vi "cvt type to tag bus type.vi"(11 "cvt type":T1) -> (3 "Data Type":T2)   [LabVIEW 2013, in "CVT configuration.lvclass"]
uses:
  CVT configuration.lvclass
  <vilib>/NI/Tag Bus/tag/Data Type.ctl
  <vilib>/NI/Current Value Table/Type Defs/Data Types.ctl
  <vilib>/NI/Tag Bus/tag/tag descriptor.lvclass
  <vilib>/NI/Current Value Table/Current Value Table.lvlib
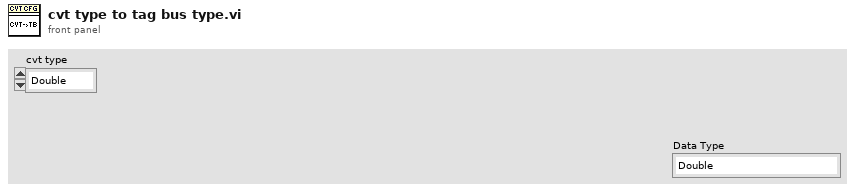
[diagram p1: front panel]
types:
  T1 = typedef "Current Value Table.lvlib/Data Types.ctl" = enum16{"Double", "Single", "I64", "I32", "I16", "I8", "U64", "U32", "U16", "U8", "String", "Boolean", "Array of U8", "Array of U16", "Array of U32", "Array of U64", "Array of I64", "Array of I32", "Array of I16", "Array of I8", "Array of Double", "Array of Single", "Array of Boolean", "Array of String"}
  T2 = typedef "tag bus.lvlib/tag descriptor.lvclass/Data Type.ctl" = enum16{"Double", "Single", "I64", "I32", "I16", "I8", "U64", "U32", "U16", "U8", "Boolean", "String", "Array of Double", "Array of Single", "Array of I64", "Array of I32", "Array of I16", "Array of I8", "Array of U64", "Array of U32", "Array of U16", "Array of U8", "Array of Boolean", "Array of String"}
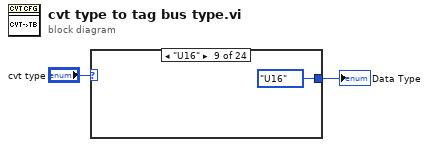
[diagram p0: block diagram]
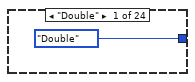
[diagram p2: hidden frame]
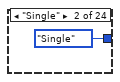
[diagram p3: hidden frame]
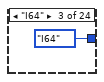
[diagram p4: hidden frame]
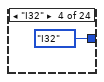
[diagram p5: hidden frame]
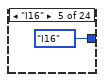
[diagram p6: hidden frame]
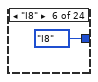
[diagram p7: hidden frame]
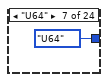
[diagram p8: hidden frame]
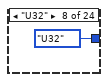
[diagram p9: hidden frame]
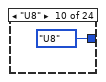
[diagram p10: hidden frame]
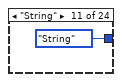
[diagram p11: hidden frame]
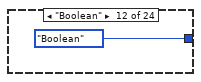
[diagram p12: hidden frame]
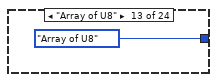
[diagram p13: hidden frame]
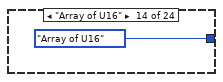
[diagram p14: hidden frame]
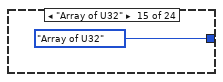
[diagram p15: hidden frame]
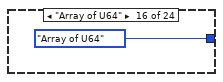
[diagram p16: hidden frame]
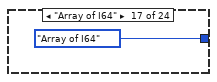
[diagram p17: hidden frame]
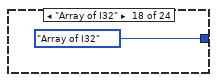
[diagram p18: hidden frame]
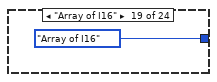
[diagram p19: hidden frame]
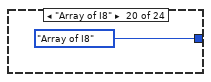
[diagram p20: hidden frame]
diagram:
  n1 = case shown="\"U16\"" "cvt type" {
    tunnel: [Data_Type."Double" ("Expected Type") Data_Type."Single" ("Expected Type") Data_Type."I64" ("Expected Type") Data_Type."I32" ("Expected Type") Data_Type."I16" ("Expected Type") Data_Type."I8" ("Expected Type") Data_Type."U64" ("Expected Type") Data_Type."U32" ("Expected Type") Data_Type."U16" ("Expected Type") Data_Type."U8" ("Expected Type") Data_Type."String" ("Expected Type") Data_Type."Boolean" ("Expected Type") Data_Type."Array of U8" ("Expected Type") Data_Type."Array of U16" ("Expected Type") Data_Type."Array of U32" ("Expected Type") Data_Type."Array of U64" ("Expected Type") Data_Type."Array of I64" ("Expected Type") Data_Type."Array of I32" ("Expected Type") Data_Type."Array of I16" ("Expected Type") Data_Type."Array of I8" ("Expected Type") Data_Type."Array of Double" ("Expected Type") Data_Type."Array of Single" ("Expected Type") Data_Type."Array of Boolean" ("Expected Type") Data_Type."Array of String" ("Expected Type")] -> w1
    frame "Double" {
    }
    frame "Single" {
    }
    frame "I64" {
    }
    frame "I32" {
    }
    frame "I16" {
    }
    frame "I8" {
    }
    frame "U64" {
    }
    frame "U32" {
    }
    frame "U16" {
    }
    frame "U8" {
    }
    frame "String" {
    }
    frame "Boolean" {
    }
    frame "Array of U8" {
    }
    frame "Array of U16" {
    }
    frame "Array of U32" {
    }
    frame "Array of U64" {
    }
    frame "Array of I64" {
    }
    frame "Array of I32" {
    }
    frame "Array of I16" {
    }
    frame "Array of I8" {
    }
    frame "Array of Double" {
    }
    frame "Array of Single" {
    }
    frame "Array of Boolean" {
    }
    frame "Array of String" {
    }
  }
  "Data Type" <- w1
